vi "Edit_States.vi"(7 "Action":T1, 8 "error in (no error)":errorcluster, 11 "MulticolumnListbox in":refnum<vi>) -> (0 "error out":errorcluster)   [LabVIEW 2016, in "Horizontal MenuList.xctl"]
uses:
  Horizontal MenuList.xctl
  Edit_Actions.ctl
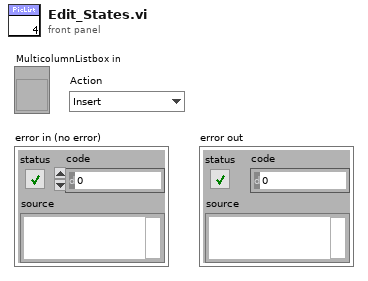
[diagram p1: front panel]
types:
  T1 = typedef "Horizontal MenuList.xctl/Edit_Actions.ctl" = enum16{"Insert", "Delete", "Move Up", "Move Down"}
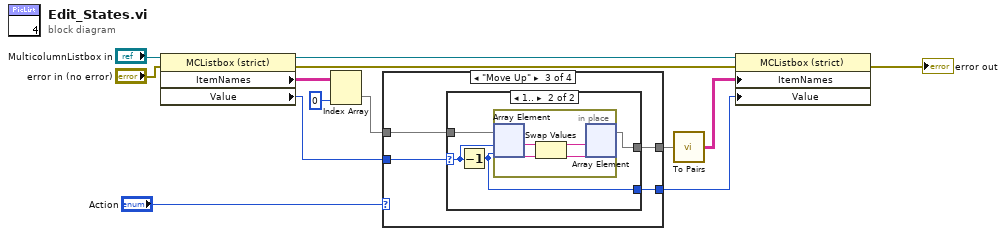
[diagram p0: block diagram]
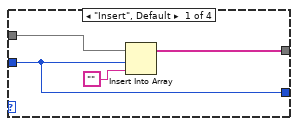
[diagram p2: hidden frame]
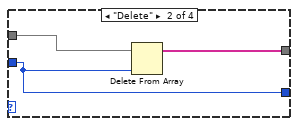
[diagram p3: hidden frame]
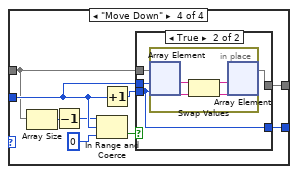
[diagram p5: hidden frame]
diagram:
  n1 = property class="MCListbox (strict)"(reference="MulticolumnListbox in", error in="error in (no error)") -> (reference out=w8:refnum<vi>, error out=w10:errorcluster, "ItemNames"=w6:string[][], "Value"=w7:i32)
  n2 = Index Array(array=w6, index (col)=0 ("disabled index (col)")) -> (element=w4:string[])  [unwired: 1 in]
  n3 = case shown="\"Move Up\"" "Action" {
    tunnel: w7 -> [w14 w18 w23 w41]
    tunnel: [w17 w19 w22 w42] -> w5
    tunnel: w4 -> [w15 w20 w24 w40]
    tunnel: [w14 w18 w21 w35] -> w1
    frame "Insert", Default {
      n4 = Insert Into Array(array=w15, index=w14, new element="") -> (w17:string[])
    }
    frame "Delete" {
      n5 = Delete From Array(array=w20, index=w18) -> (array with subset deleted=w19:string[])  [unwired: 1 in, 1 out]
    }
    frame "Move Up" {
      n6 = case shown="1.." w23 {
        selector: w23 -> [w25 w29]
        tunnel: w24 -> [w26 w30]
        tunnel: [w26 w28] -> w22
        tunnel: [w25 w27] -> w21
        frame 0, Default {
        }
        frame 1.. {
          n7 = Decrement(x=w29) -> (x-1=w27:i32)
          n8 = in-place {
            n9 = in-place-array #1(w30, w29, w27) -> (w34:string, w33:string)
            n10 = Swap Values(12:w34, 14:w33) -> (1:w32:string, 3:w31:string)  [unwired: 1 in]
            n11 = in-place-array #1(w32, w31) -> (w28:string[])  [unwired: 2 out]
          }
        }
      }
    }
    frame "Move Down" {
      n12 = Array Size(array=w40) -> (size(s)=w39:i32)
      n13 = Decrement(x=w39) -> (x-1=w38:i32)
      n14 = In Range and Coerce(upper limit=w38, x=w41, lower limit=0) -> (In Range?=w36:bool)  [unwired: 1 out]
      n15 = Increment(x=w41) -> (x+1=w43:i32)
      n16 = case shown="True" w36 {
        tunnel: w43 -> [_ w46]
        tunnel: [w45 w49] -> w42
        tunnel: w41 -> [w44 w48]
        tunnel: w40 -> [w45 w47]
        tunnel: [w44 w46] -> w35
        frame False {
        }
        frame True {
          n17 = in-place {
            n18 = in-place-array #2(w47, w48, w46) -> (w53:string, w52:string)
            n19 = Swap Values(12:w53, 14:w52) -> (1:w51:string, 3:w50:string)  [unwired: 1 in]
            n20 = in-place-array #2(w51, w50) -> (w49:string[])  [unwired: 2 out]
          }
        }
      }
    }
  }
  n21 = call "To Pairs.vi"("Elements"=w5) -> ("Array"=w9:string[][])  [unwired: 4 in]
  n22 = property class="MCListbox (strict)"(reference=w8, error in=w10, "ItemNames"=w9, "Value"=w1) -> (error out=→"error out":errorcluster)  [unwired: 1 out]
